vi "Get Pinmap Client.vi"(8 "error in (no error)":errorcluster, 11 "ClientPool in":refnum<class "ClientPool.lvclass">) -> (0 "error out":errorcluster, 2 "Pinmap grpc id":T1, 3 "ClientPool out":refnum<class "ClientPool.lvclass">)   [LabVIEW 2020, in "MeasurementLink Measurement Server.lvlib" / "ClientPool.lvclass"]
uses:
  ClientPool.lvclass
  <vilib>/gRPC/LabVIEW gRPC Library/Shared/grpcId.ctl
  ClientPool.lvclass/ClientPool.ctl
  MeasurementLink Discovery Client/RPC Messages/ni_measurementlink_discovery_v1_ResolveServiceRequest.ctl
  MeasurementLink Discovery Client/MeasurementLink Discovery Client.lvlib
  MeasurementLink Pin Map Client/MeasurementLink Pin Map Client.lvlib
  <vilib>/gRPC/LabVIEW gRPC Library/grpc-lvsupport-release.lvlib
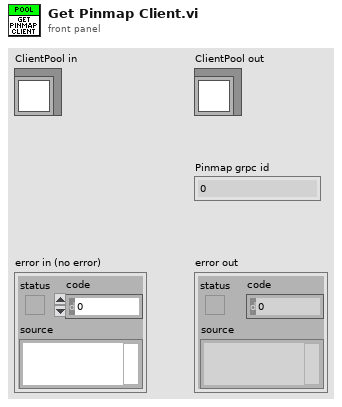
[diagram p1: front panel]
types:
  T1 = typedef "grpc-lvsupport-release.lvlib/grpcId.ctl" = u64
  T2 = typedef "MeasurementLink Discovery Client.lvlib/ni_measurementlink_discovery_v1_ResolveServiceRequest.ctl" = cluster{"provided_interface":string, "service_class":string}
  T3 = typedef "MeasurementLink Discovery Client.lvlib/ni_measurementlink_discovery_v1_ServiceLocation.ctl" = cluster{"location":string, "insecure_port":string, "ssl_authenticated_port":string}
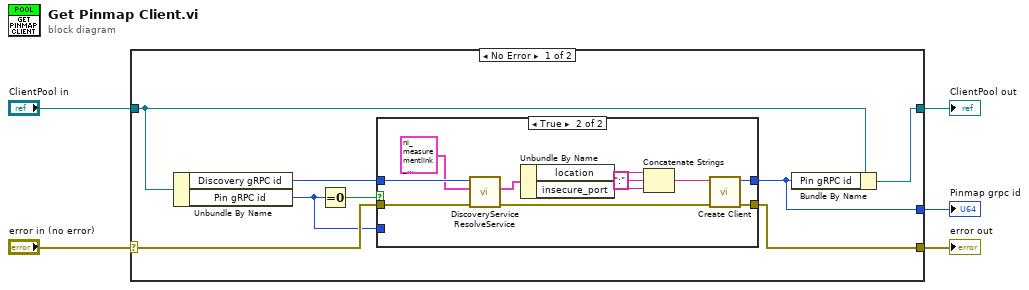
[diagram p0: block diagram]
diagram:
  n1 = case shown="No Error" "error in (no error)" {
    selector: "error in (no error)" -> [w11 w28]
    tunnel: [w10 w28] -> w4
    tunnel: [w7 w27] -> w2
    tunnel: "ClientPool in" -> [w8 w27]
    tunnel: [w6 _] -> w1
    frame No Error {
      n2 = Unbundle By Name(w8) -> ("Discovery gRPC id"=w12:T1, "Pin gRPC id"=w9:T1)
      n3 = Equal To 0?(x=w9) -> (x = 0?=w13:bool)
      n4 = case shown="True" w13 {
        tunnel: w12 -> [_ w20]
        tunnel: w11 -> [w15 w19]
        tunnel: [w14 w18] -> w6
        tunnel: [w15 w17] -> w10
        tunnel: w9 -> [w14 _]
        frame False {
        }
        frame True {
          n5 = call "DiscoveryService ResolveService.vi"("error in"=w19, "Request Data"=T2 {"provided_interface"="ni.measurementlink.pinmap.v1.PinMapService", "service_class"="ni.measurementlink.pinmap.v1.PinMapService"}, "gRPC ID"=w20) -> ("error out"=w21:errorcluster, "Response Data"=w26:T3)  [unwired: 6 in, 1 out]
          n6 = Unbundle By Name(w26) -> ("location"=w25:string, "insecure_port"=w24:string)
          n7 = Concatenate Strings(w25, ":" ("string"), w24) -> (w22:string)
          n8 = call "Create Client.vi"("error in"=w21, "address"=w22) -> ("error out"=w17:errorcluster, "gRPC ID Out"=w18:T1)  [unwired: 8 in]
        }
      }
      n9 = Bundle By Name(cluster=w8, "Pin gRPC id"=w6) -> (w7:refnum<class "ClientPool.lvclass">)
    }
    frame Error {
    }
  }
  "error out" <- w4
  "ClientPool out" <- w2
  "Pinmap grpc id" <- w1
